vi "StopSignal-GenerateInOrder.vi"(8 "error in (no error)":errorcluster, 9 "interval time(ms)":u32, 10 "reason(\"\")":string, 11 "name(\"\")":string[](array[string])) -> (0 "error out":errorcluster)   [LabVIEW 2017, in "StopSignal.lvlib"]
uses:
  StopSignal.lvlib
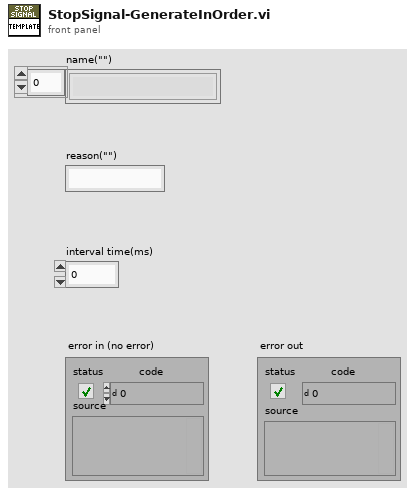
[diagram p1: front panel]
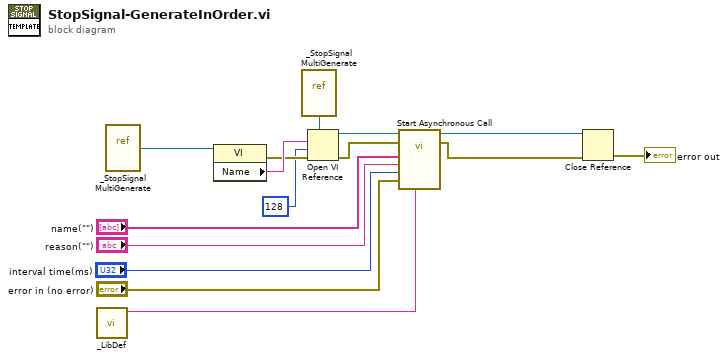
[diagram p0: block diagram]
diagram:
  n1 = call "_LibDef.vi"() -> ("LIBNAME"=w2:string)  [unwired: 11 in]
  n2 = vi-ref "_StopSignal MultiGenerate.vi"() -> (w13:refnum<vi>)
  n3 = property class="VI"(reference=w13) -> (error out=w14:errorcluster, "Name"=w15:string)  [unwired: 1 in, 1 out]
  n4 = vi-ref "_StopSignal MultiGenerate.vi"() -> (w12:refnum<vi>)
  n5 = Open VI Reference(type specifier VI Refnum (for type only)=w12, vi path=w15, options=128, error in (no error)=w14) -> (vi reference=w11:refnum<vi>, error out=w10:errorcluster)  [unwired: 2 in]
  n6 = call-by-ref "Start Asynchronous Call"(reference=w11, error in=w10, "LIBNAME"=w2, 8:"error in (no error)"="error in (no error)", "interval time(ms)"="interval time(ms)", "reason(\"\")"="reason(\"\")", "name(\"\")"="name(\"\")") -> (reference out=w8:refnum<vi>, error out=w9:errorcluster)  [unwired: 5 in, 2 out]
  n7 = Close Reference(reference=w8, error in (no error)=w9) -> (error out=→"error out":errorcluster)
